vi "respond to response.vi"(8 "error in (no error)":errorcluster caption="Fehler (Eingang, kein Fehler)", 10 "?":T1={"commandlist"="", "line"=0, "last response"="", "timeout"=0, "wait"=0, "erfolgreich"=FALSE, "next state"=enum."init", "Zustand"=enum."starting", "manual Test"=FALSE}, 11 "TestInterface Eingang":refnum<class "TestInterface.lvclass"> caption="DNL_LabVIEW Object in") -> (0 "error out":errorcluster caption="Fehler (Ausgang)", 1 "read again?":bool, 2 "Cluster":T1={"commandlist"="", "line"=0, "last response"="", "timeout"=0, "wait"=0, "erfolgreich"=FALSE, "next state"=enum."init", "Zustand"=enum."starting", "manual Test"=FALSE}, 3 "TestInterface Ausgang":refnum<class "TestInterface.lvclass"> caption="DNL_LabVIEW Object out")   [LabVIEW 2013, in "TestInterface.lvclass"]
doc: "In diesem VI wird auch der aktuelle Befehl inspiziert. Allerdings wird zusätzlich die empfangene Antwort angeschaut. Sollte die Antwort nicht der Erwartung entsprechen, kann auf den Programmablauf Einfluss genommen werden, indem die Kommandoliste verändert wird. Dies ist besonders sinnvoll, wenn ein Gerät gefragt wird, ob es bereits mit dem aktuellen Test fertig ist. Sollte das Gerät dies verneinen, kann nach einer Weile eine neue Anfrage gestellt werden. Dies wird so lange wiederholt, bis der Test abgeschlossen ist."
uses:
  TestInterface.lvclass
  Main/controls/TestData.ctl
  Main/controls/TestStates.ctl
  Main/controls/generalTestStates.ctl
  lib/EMV-Test.lvlib
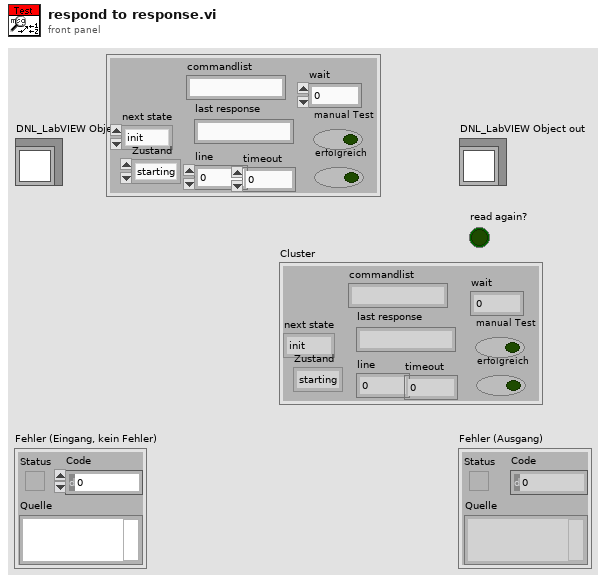
[diagram p1: front panel]
types:
  T1 = typedef "EMV-Test.lvlib/TestData.ctl" = cluster{"commandlist":string, "line":i32, "last response":string, "timeout":i32, "wait":u32, "erfolgreich":bool, "next state":T2, "Zustand":T3, "manual Test":bool}
  T2 = typedef "EMV-Test.lvlib/TestStates.ctl" = enum16{"event loop", "save Test", "Custom Action 1", "Custom Action 2", "pause", "vorgefertigter Test", "manueller Test", "respond to response", "error", "init", "start Test", "evaluate line", "wait for Response", "wait", "catch error", "close Connection", "end"}
  T3 = typedef "generalTestStates.ctl" = enum16{"paused", "starting", "waiting", "running", "finished"}
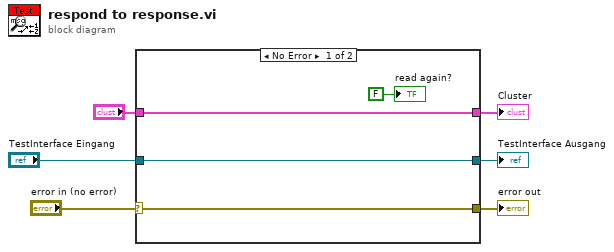
[diagram p0: block diagram]
diagram:
  n1 = case shown="No Error" "error in (no error)" {
    selector: "error in (no error)" -> [w9 w13]
    tunnel: [w9 w13] -> w5
    tunnel: [w10 w12] -> w3
    tunnel: "TestInterface Eingang" -> [w10 w12]
    tunnel: [w8 w11] -> w1
    tunnel: "?" -> [w8 w11]
    frame No Error {
      "read again?" <- FALSE ("read again?")
    }
    frame Error {
    }
  }
  "error out" <- w5
  "TestInterface Ausgang" <- w3
  "Cluster" <- w1
